vi "movment estimate.vi"(0 "speed array in":dbl[](array[numeric]), 5 "speed":dbl, 7 "start":bool, 9 "speed limit change":dbl=0.05 format="%#_13g") -> (4 "total movement":dbl, 6 "speed array out":dbl[](array[numeric]))   [LabVIEW 2019]
panel:
  out "previous movment":dbl
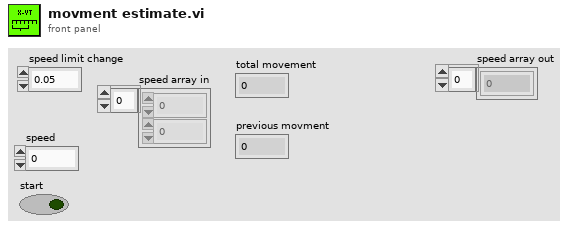
[diagram p1: front panel]
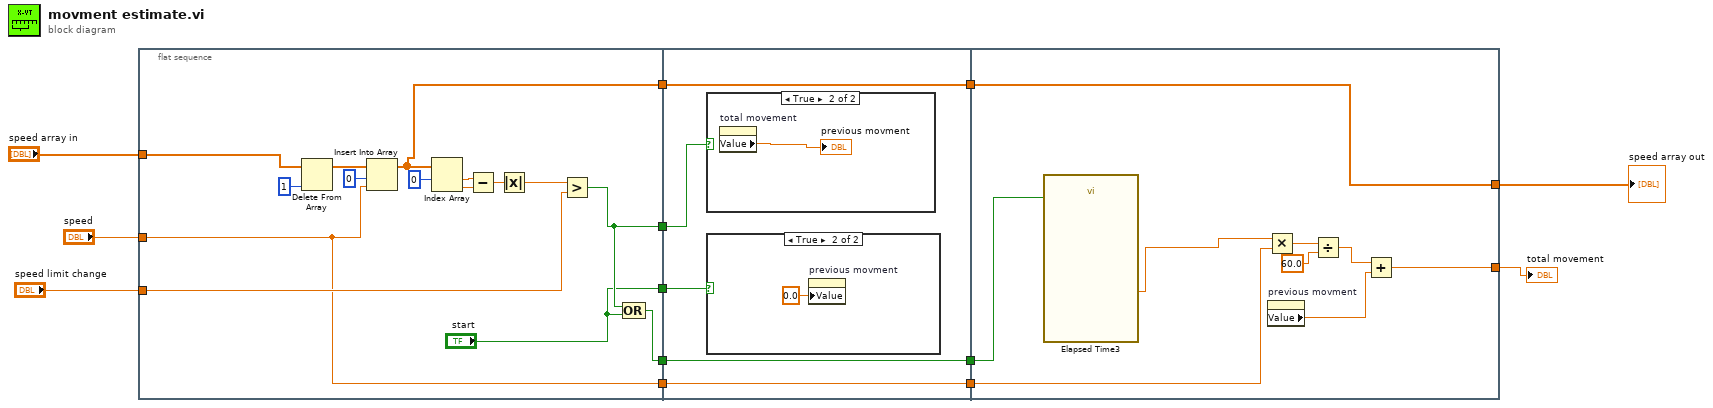
[diagram p0: block diagram]
diagram:
  n1 = flat-sequence {
    tunnel: "speed array in" -> [w20]
    tunnel: "speed" -> [w15]
    tunnel: "speed limit change" -> [w19]
    tunnel: [w17] -> w9
    tunnel: [w18] -> w8
    tunnel: ["start"] -> w7
    tunnel: [w15] -> w5
    tunnel: [w14] -> w2
    tunnel: [w33] -> w10
    tunnel: w9 -> [w33]
    tunnel: w8 -> [w32]
    tunnel: w7 -> [w31]
    tunnel: [w30] -> w6
    tunnel: w5 -> [w30]
    tunnel: [w29] -> w3
    tunnel: w2 -> [w29]
    tunnel: w10 -> [w44]
    tunnel: w6 -> [w38]
    tunnel: [w37] -> w4
    tunnel: w3 -> [w36]
    tunnel: [w36] -> w1
    frame #0 {
      n2 = Delete From Array(array=w20, index=1) -> (array with subset deleted=w26:dbl[])  [unwired: 1 in, 1 out]
      n3 = Insert Into Array(array=w26, index=0, new element=w15) -> (w14:dbl[])
      n4 = Index Array(array=w14, index #1=0 ("index")) -> (element #1=w27:dbl, element #2=w28:dbl)  [unwired: 1 in]
      n5 = Subtract(x=w27, y=w28) -> (x-y=w23:dbl)
      n6 = Absolute Value(x=w23) -> (abs(x)=w22:dbl)
      n7 = Greater?(x=w22, y=w19) -> (0:w18:bool)
      n8 = Compound Arithmetic op=OR(w18, "start") -> (w17:bool)
    }
    frame #1 {
      n9 = case shown="True" w32 {
        frame False {
        }
        frame True {
          n10 = property on="total movement" class="DigNum (strict)"() -> ("Value"=→"previous movment":dbl)  [unwired: 2 in, 2 out]
        }
      }
      n11 = case shown="True" w31 {
        frame False {
        }
        frame True {
          n12 = property on="previous movment" class="DigNum (strict)"("Value"=0.0 ("previous movment")) -> ()  [unwired: 2 in, 2 out]
        }
      }
    }
    frame #2 {
      n13 = call "Elapsed Time3"("Reset"=w44) -> ("Elapsed Time (s)"=w39:dbl)  [unwired: 11 in, 7 out]
      n14 = Multiply(x=w39, y=w38) -> (x*y=w40:dbl)
      n15 = property on="previous movment" class="DigNum (strict)"() -> ("Value"=w43:dbl)  [unwired: 2 in, 2 out]
      n16 = Divide(x=w40, y=60.0) -> (x/y=w42:dbl)
      n17 = Add(x=w42, y=w43) -> (x+y=w37:dbl)
    }
  }
  "speed array out" <- w1
  "total movement" <- w4
